vi "testqrcode.vi"() -> ()   [LabVIEW 2019]
uses:
  <vilib>/vision/Instrument.llb/QR Code Report.ctl
  <vilib>/vision/Instrument.llb/QR Code Model Type.ctl
  <vilib>/vision/Instrument.llb/QR Code Stream Mode Type.ctl
  <vilib>/vision/Instrument.llb/Data Matrix Polarity.ctl
  <vilib>/vision/Instrument.llb/Demodulation Mode.ctl
  <vilib>/vision/Instrument.llb/Cell Sample Size.ctl
  <vilib>/vision/Instrument.llb/Cell Filter Mode.ctl
panel:
  out "Number of Particles (Particle Analysis 1)":i32
  out "Particle Measurements (Pixels) (Particle Analysis 1)":dbl[][](array[numeric]) format="%.2f"
  out "Image":T1(plugin-control)
  out "QR Barcode Report (2D Barcode Reader 1)":T2={"Found?"=FALSE, "Data"="", "Bounding Box"=[], "Errors Corrected"=0, "Dimensions (Rows/Cols)"=0, "Version"=0, "QR Model"=3, "Stream Mode"=0, "Barcode Polarity"=-2, "Mirrored?"=FALSE, "Append Stream Position"=0, "Size of Append Stream"=0, "First EAN-128 ID"=0, "First Alternate Language ID"=0, "Append Stream ID"=0, "Minimum Edge Strength"=30, "Demodulation Mode"=-2, "Cell Sample Size"=-2, "Cell Filter Mode"=-2} {"Append Stream ID" format="%x"; "Cell Filter Mode" items=["Auto-detect"=-2, "Average"=0, "Median"=1, "Central Average"=2, "High Average"=3, "Low Average"=4, "Very High Average"=5, "Very Low Average"=6, "All Filters"=8]; "Cell Sample Size" items=["Auto-detect"=-2, "1x1"=1, "2x2"=2, "3x3"=3, "4x4"=4, "5x5"=5, "6x6"=6, "7x7"=7]; "Demodulation Mode" items=["Auto-detect"=-2, "Histogram"=0, "Local Contrast"=1, "Combination"=2, "All"=3]; "Barcode Polarity" items=["Auto-detect"=-2, "Black on White"=0, "White on Black"=1]; "Stream Mode" items=["Auto-detect", "Numeric", "AlphaNumeric", "Mixed", "Raw Bytes", "UCC/EAN-128 - In Tokens", "UCC/EAN-128 - In Data", "Extended Character Interpretation", "Kanji"]; "QR Model" items=["Auto Detect", "Micro", "Model 1", "Model 2"]; "Version" max=40 step=1}
  in  "Zoom::Value":i64 min=0 max=10 step=1
  in  "Stop (F)":bool
  out "Image Out":T1(plugin-control)
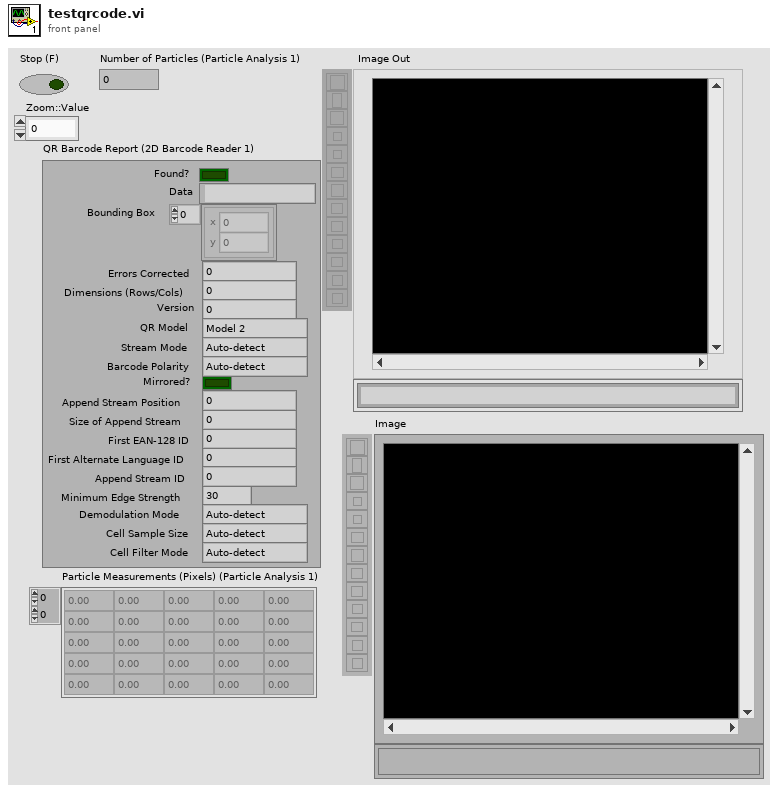
[diagram p1: front panel]
types:
  T1 = typedef "IMAQ Image.ctl" = refnum<image>
  T2 = typedef "QR Code Report.ctl" = cluster{"Found?":bool, "Data":string, "Bounding Box":cluster{"x":sgl, "y":sgl}[], "Errors Corrected":u32, "Dimensions (Rows/Cols)":u32, "Version":u32, "QR Model":T3, "Stream Mode":T4, "Barcode Polarity":T5, "Mirrored?":bool, "Append Stream Position":u32, "Size of Append Stream":u32, "First EAN-128 ID":i32, "First Alternate Language ID":i32, "Append Stream ID":u32, "Minimum Edge Strength":u32, "Demodulation Mode":T6, "Cell Sample Size":T7, "Cell Filter Mode":T8}
  T3 = typedef "QR Code Model Type.ctl" = i32
  T4 = typedef "QR Code Stream Mode Type.ctl" = i32
  T5 = typedef "Data Matrix Polarity.ctl" = i32
  T6 = typedef "Demodulation Mode.ctl" = i32
  T7 = typedef "Cell Sample Size.ctl" = i32
  T8 = typedef "Cell Filter Mode.ctl" = i32
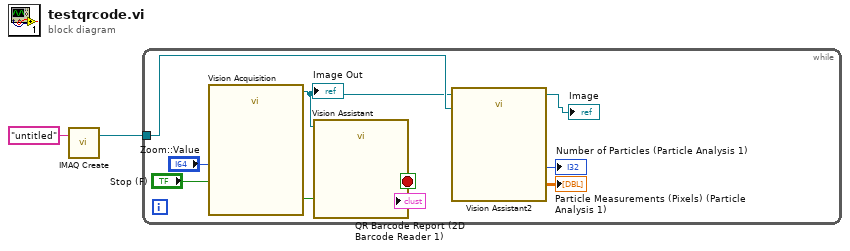
[diagram p0: block diagram]
diagram:
  n1 = call "IMAQ Create"("Image Name"="untitled") -> ("New Image"=w1:T1)  [unwired: 4 in, 1 out]
  n2 = while {
    tunnel: w1 -> [w7]
    stop <- w10 stop-if-true
    n3 = call "Vision Acquisition"("Zoom::Value"="Zoom::Value", "Stop (F)"="Stop (F)") -> ("Image Out"=w5:T1, "Stopped"=w10:bool)  [unwired: 23 in, 1 out]
    "Image Out" <- w5
    n4 = call "Vision Assistant"("Image In"=w5) -> ("QR Barcode Report (2D Barcode Reader 1)"=→"QR Barcode Report (2D Barcode Reader 1)":T2)  [unwired: 24 in, 2 out]
    n5 = call "Vision Assistant2"("Image In"=w5, "Image Dst"=w7) -> ("Image Out"=→"Image":T1, "Number of Particles (Particle Analysis 1)"=→"Number of Particles (Particle Analysis 1)":i32, "Particle Measurements (Pixels) (Particle Analysis 1)"=→"Particle Measurements (Pixels) (Particle Analysis 1)":dbl[][])  [unwired: 22 in, 1 out]
  }
